vi "test 3- normalModeCallsWorkerMode.vi"(8 "error in (no error)":errorcluster, 11 "TestCase in":refnum<class "testcase-SyncMessage.lvclass">) -> (0 "error out":errorcluster, 3 "TestCase out":refnum<class "testcase-SyncMessage.lvclass">)   [LabVIEW 2017, in "testcase-SyncMessage.lvclass"]
uses:
  testcase-SyncMessage.lvclass
  <vilib>/addons/_JKI Toolkits/VI Tester/TestCase.llb/TestCase.lvclass
  src/user.lib/_NEVSTOP/Communicable State Machine(CSM)/Communicable State Machine.lvlib
  C:/Program Files (x86)/National Instruments/LabVIEW 2017/vi.lib/addons/_JKI Toolkits/VI Tester/TestCase.llb/TestCase.lvclass
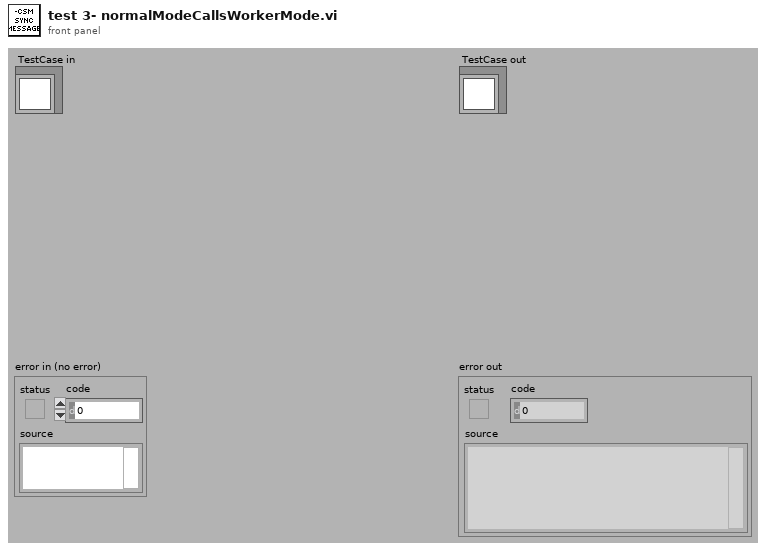
[diagram p1: front panel]
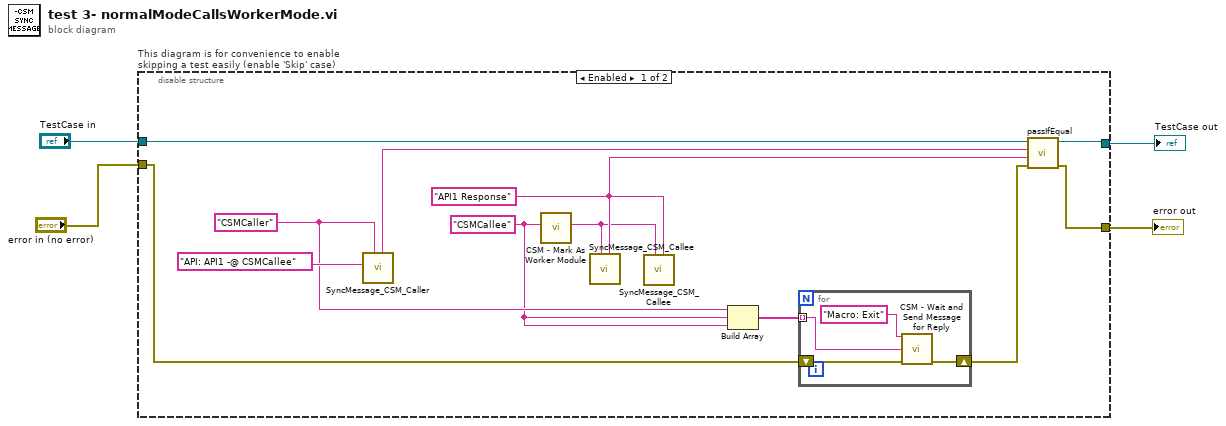
[diagram p0: block diagram]
diagram:
  n1 = disable-structure "This diagram is for convenience to enable skipping a test easily (enable 'Skip' case)" shown="Enabled" {
    disable-tunnel: "TestCase in" -> [w16 w24]
    disable-tunnel: [w15 w22] -> w2
    disable-tunnel: [w14 w23] -> w1
    disable-tunnel: "error in (no error)" -> [w5 w21]
    frame Enabled {
      w6 = "CSMCallee" ("CSMCallee")
      w10 = "CSMCaller" ("CSMCaller")
      w8 = "API1 Response" ("API response in")
      n2 = call "SyncMessage_CSM_Caller.vi"("Name (\"\" to Use UUID)"=w10, "Intermodule Message in"="API: API1 -@ CSMCallee") -> ("API received Response out"=w12:string)  [unwired: 9 in]
      n3 = call "CSM - Mark As Worker Module.vi"("CSM Name"=w6) -> ("CSM Name (Marked As Worker)"=w7:string)  [unwired: 9 in]
      n4 = call "SyncMessage_CSM_Callee.vi"("API response in"=w8, "Name (\"\" to Use UUID)"=w7) -> ()  [unwired: 10 in]
      n5 = call "SyncMessage_CSM_Callee.vi"("API response in"=w8, "Name (\"\" to Use UUID)"=w7) -> ()  [unwired: 10 in]
      n6 = Build Array(w10, w6, w6) -> (w11:string[])
      n7 = for {
        shift-right: [w18] -> w9
        shift-left: w5 -> [w19]
        tunnel: w11 -> [w17] mode=indexing
        n8 = call "CSM - Wait and Send Message for Reply.vi"("State"="Macro: Exit", "Target Module"=w17, "Error In (No Error)"=w19) -> ("error out"=w18:errorcluster)  [unwired: 10 in, 2 out]
      }
      n9 = call-dynamic "passIfEqual.vi"("error in (no error)"=w9, "y"=w8, "x"=w12, "TestCase in"=w16) -> ("error out"=w14:errorcluster, "TestCase out"=w15:refnum<class "testcase-SyncMessage.lvclass">)  [unwired: 6 in]
    }
    frame Disabled {
      # "skip test result while test is under development"
      n10 = call <vilib>:"skip.vi"("error in (no error)"=w21, "TestCase in"=w24) -> ("error out"=w23:errorcluster, "TestCase out"=w22:refnum<class "testcase-SyncMessage.lvclass">)  [unwired: 8 in]
    }
  }
  "error out" <- w1
  "TestCase out" <- w2
